vi "Asynchronous Find Systems.vi"(10 "Find Systems Configuration":T1={"Session in (localhost)"="localhost", "Device Class"="", "Detect Online Systems (T)"=TRUE, "Include Cached Results (all)"=3, "Output (Hostname and IP)"=18, "Timeout (4000 ms)"=4000, "Only Installable Systems (F)"=FALSE} {"Output (Hostname and IP)" items=["Hostname"=16, "Hostname (IP)"=18, "Hostname (MAC)"=19, "IP"=32, "IP (Hostname)"=33, "IP (MAC)"=35, "MAC"=48, "MAC (Hostname)"=49, "MAC (IP)"=50]; "Include Cached Results (all)" items=["none"=0, "only if online"=1, "all"=3]}, 11 "Queue reference":refnum<queue>) -> ()   [LabVIEW 2015]
uses:
  Controls/FindSystemsConfiguration.ctl
  <vilib>/nisyscfg/nisyscfg.lvlib
  RT Management.lvclass
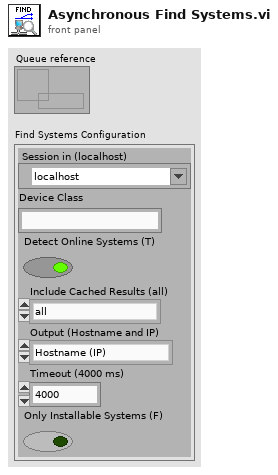
[diagram p1: front panel]
types:
  T1 = typedef "RT Management.lvlib/RT Management.lvclass/FindSystemsConfiguration.ctl" = cluster{"Session in (localhost)":refnum<k21>, "Device Class":string, "Detect Online Systems (T)":bool, "Include Cached Results (all)":u32, "Output (Hostname and IP)":u32, "Timeout (4000 ms)":u32, "Only Installable Systems (F)":bool}
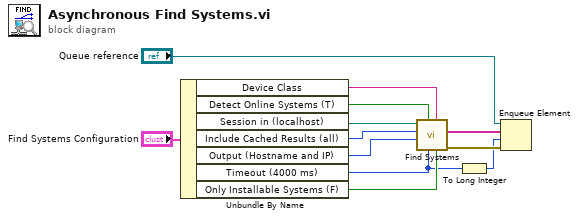
[diagram p0: block diagram]
diagram:
  n1 = Unbundle By Name("Find Systems Configuration") -> ("Device Class"=w11:string, "Detect Online Systems (T)"=w10:bool, "Session in (localhost)"=w9:refnum<k21>, "Include Cached Results (all)"=w8:u32, "Output (Hostname and IP)"=w7:u32, "Timeout (4000 ms)"=w2:u32, "Only Installable Systems (F)"=w6:bool)
  n2 = call <vilib>:"Find Systems.vi"("Only Installable Systems (F)"=w6, "Device Class"=w11, "Timeout (4000 ms)"=w2, "Detect Online Systems (T)"=w10, "Output (Hostname and IP)"=w7, "Include Cached Results (all)"=w8, "Session in (localhost)"=w9) -> ("error out"=w5:errorcluster, "Detected Systems"=w3:string[])  [unwired: 2 in, 1 out]
  n3 = To Long Integer(number=w2) -> (32bit integer=w1:i32)
  n4 = Enqueue Element(queue="Queue reference", element=w3, timeout in ms (-1)=w1, error in (no error)=w5) -> ()  [unwired: 3 out]
